vi "getIntegrationTime.vi"(8 "error in (no error)":errorcluster, 11 "Electrometer in":refnum<class "Electrometer.lvclass">) -> (0 "error out":errorcluster, 3 "Electrometer out":refnum<class "Electrometer.lvclass">)   [LabVIEW 2016, in "Electrometer.lvclass"]
uses:
  Electrometer.lvclass
  Modes.ctl
panel:
  out "Integration Time":string
  in  "Measurement Function (0: Current)":T1
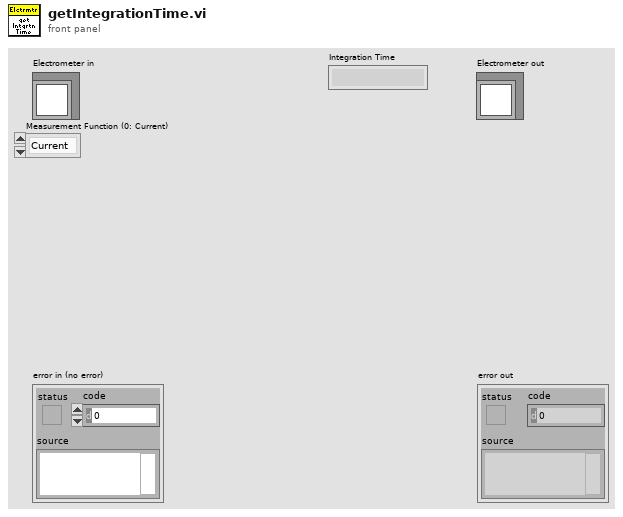
[diagram p1: front panel]
types:
  T1 = typedef "Electrometer.lvclass/Modes.ctl" = enum16{"Current", "Charge", "Voltage", "Resistance"}
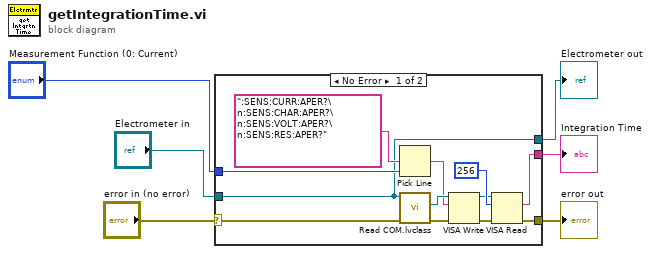
[diagram p0: block diagram]
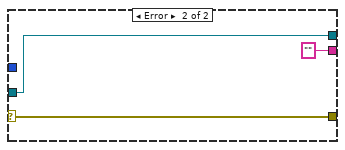
[diagram p2: hidden frame]
diagram:
  n1 = case shown="No Error" "error in (no error)" {
    selector: "error in (no error)" -> [w12 w21]
    tunnel: [w8 w21] -> w5
    tunnel: [w13 w20] -> w3
    tunnel: "Electrometer in" -> [w13 w20]
    tunnel: "Measurement Function (0: Current)" -> [w17 _]
    tunnel: [w7 "" ("read buffer")] -> w1
    frame No Error {
      n2 = Pick Line(multi-line string=":SENS:CURR:APER?\n:SENS:CHAR:APER?\n:SENS:VOLT:APER?\n:SENS:RES:APER?", line index=w17) -> (output string=w14:string)  [unwired: 1 in]
      n3 = call "Read COM.lvclass.vi"("error in (no error)"=w12, "Electrometer in"=w13) -> ("error out"=w16:errorcluster, "VISA"=w15:refnum<visa-resource-name>)  [unwired: 7 in, 1 out]
      n4 = VISA Write(VISA resource name=w15, write buffer=w14, error in (no error)=w16) -> (VISA resource name out=w10:refnum<visa-resource-name>, error out=w9:errorcluster)  [unwired: 1 out]
      n5 = VISA Read(VISA resource name=w10, byte count=u32 256, error in (no error)=w9) -> (read buffer=w7:string, error out=w8:errorcluster)  [unwired: 2 out]
    }
    frame Error {
    }
  }
  "error out" <- w5
  "Electrometer out" <- w3
  "Integration Time" <- w1
